vi "Module Multiply.vi"(7 "channel":T1, 10 "self":string, 11 "caller":string) -> ()   [LabVIEW 2020]
uses:
  59e6339f-7942-4da7-9608-513ec9795496.vi
  c1a7a8bb-78bf-4a95-8c01-4019f4d0a952.vi
  <extravilib>/ChannelInstances/Event MessengerM-c(str,var)/))Channel.ctl
  <extravilib>/ChannelInstances/Event MessengerM-c(str,var).lvlib
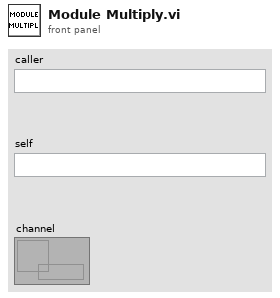
[diagram p1: front panel]
types:
  T1 = typedef "Event MessengerM-c(str,var).lvlib/))Channel.ctl" = refnum<queue>
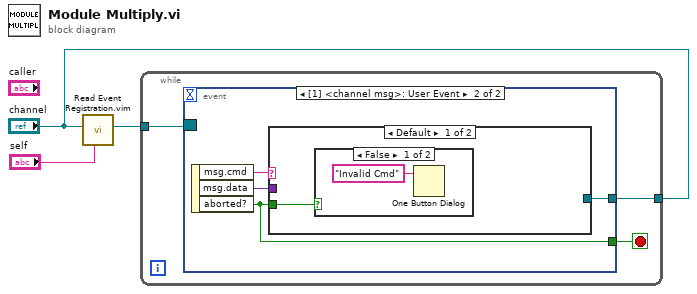
[diagram p0: block diagram]
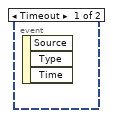
[diagram p2: hidden frame]
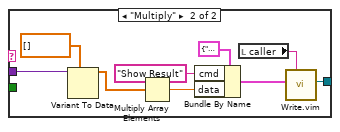
[diagram p4: hidden frame]
diagram:
  n1 = call "Read Event Registration.vim"("subchannel"="self", "channel"="channel") -> ("event registration refnum"=w3:refnum<event-registration>)  [unwired: 9 in]
  n2 = while {
    tunnel: w3 -> [w6]
    tunnel: "channel" -> [w4]
    stop <- w5 stop-if-true
    n3 = event shown="[1] <channel msg>: User Event" {
      selector: w6 -> [_ _]
      dyn-events: _ -> [_ _]
      timeout: _ -> [_ _]
      tunnel: [_ w7] -> w5
      tunnel: [_ w8] -> w4
      event Timeout {
        n4 = event-data() -> ()  [unwired: 1 in, 3 out]
      }
      event User Event {
        n5 = event-data() -> ("msg.cmd"=w10:string, "msg.data"=w9:variant, "aborted?"=w7:bool)  [unwired: 1 in]
        n6 = case shown="Default" w10 {
          tunnel: w9 -> [_ w18]
          tunnel: [_ w14] -> w8
          tunnel: w7 -> [w11 _]
          frame Default {
            n7 = case shown="False" w11 {
              frame False {
                n8 = One Button Dialog(message="Invalid Cmd") -> ()  [unwired: 1 in, 1 out]
              }
              frame True {
              }
            }
          }
          frame "Multiply" {
            n9 = Variant To Data(type=dbl[] [], Variant=w18) -> (data=w16:dbl[])  [unwired: 1 in, 1 out]
            n10 = Multiply Array Elements(1:w16) -> (0:w13:dbl)
            n11 = Bundle By Name(cluster=cluster{"cmd":string, "data":variant} {"cmd"="Show Result", "data"=variant}, "cmd"="Show Result", "data"=w13) -> (w21:cluster{"cmd":string, "data":variant})
            n12 = local read "caller"() -> (w15:string)
            n13 = call "Write.vim"("subchannel"=w15, "element"=w21) -> ("channel"=w14:T1)  [unwired: 8 in, 1 out]
          }
        }
      }
    }
  }
